vi "S8300E_BARCODE.vi"() -> ()   [LabVIEW 2011]
uses:
  <vilib>/event_ctls.llb/eventvkey.ctl
panel:
  out "軟體版本Software Version":string
  out "begin":u32
  in  "Product SN產品序號":string="192.168.1.3\n192.168.1.1\n192.168.1.1"
  # "輸入條碼上的資訊"
  # "2014-8-21"
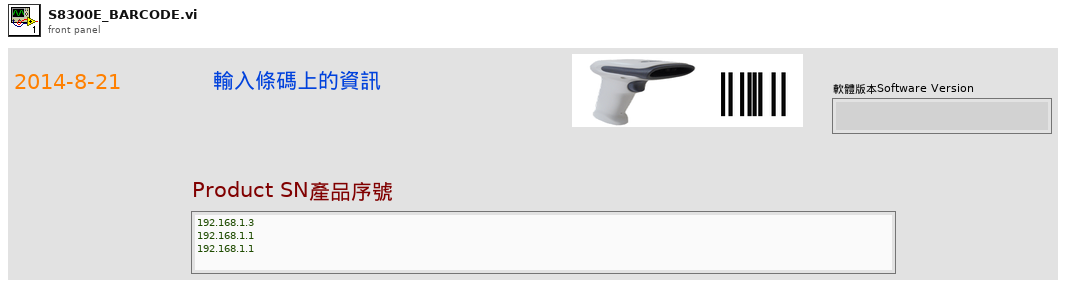
[diagram p1: front panel]
types:
  T1 = typedef "eventvkey.ctl" = enum16{"ASCII", "Enter", "Return", "Shift", "Ctrl", "Alt", "Cmd", "Opt", "Caps", "NumLock", "Clear", "Break", "Up", "Down", "Left", "Right", "Insert", "Delete", "Home", "End", "PageUp", "PageDown", "Escape", "Help", "Pause", "ScrollLock", "F1", "F2", "F3", "F4", "F5", "F6", "F7", "F8", "F9", "F10", "F11", "F12", "F13", "F14", "F15", "F16", "F17", "F18", "F19", "F20", "F21", "F22", "F23", "F24", "Play", "VolumeUp", "VolumeDown", "Mute", "Two Byte Char"}
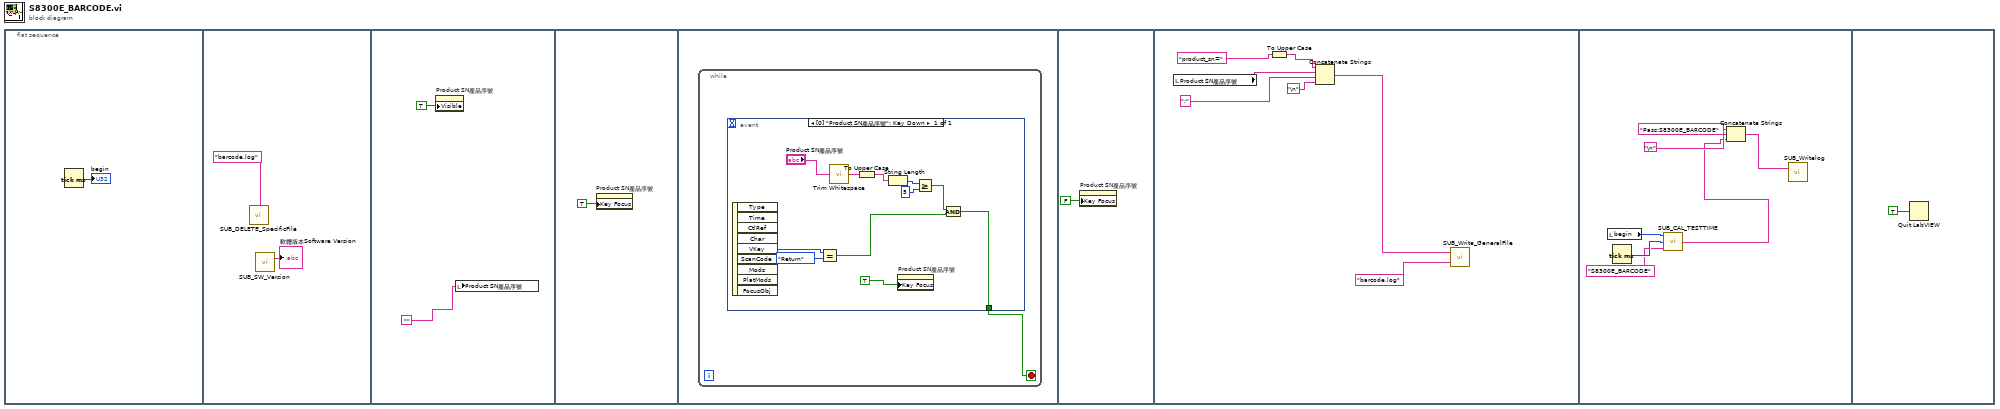
[diagram p0: block diagram]
diagram:
  n1 = flat-sequence {
    frame #0 {
      n2 = Tick Count (ms)() -> (millisecond timer value=→"begin":u32)
    }
    frame #1 {
      n3 = call "SUB_DELETE_SpecificFile.vi"("Filename to be  Deleted"="barcode.log" ("Filename")) -> ()  [unwired: 2 in, 1 out]
      n4 = call "SUB_SW_Version.vi"() -> ("Current Software Version"=→"軟體版本Software Version":string)  [unwired: 3 in]
    }
    frame #2 {
      n5 = property on="Product SN產品序號" class="Str"("Visible"=TRUE) -> ()  [unwired: 2 in, 2 out]
      n6 = local write "Product SN產品序號"("") -> ()
    }
    frame #3 {
      n7 = property on="Product SN產品序號" class="Str"("Key Focus"=TRUE) -> ()  [unwired: 2 in, 2 out]
    }
    frame #4 {
      n8 = while {
        stop <- w7 stop-if-true
        n9 = event shown="[0] \"Product SN產品序號\": Key Down" {
          selector: _ -> [_]
          dyn-events: _ -> [_]
          timeout: _ -> [_]
          tunnel: [w9] -> w7
          event "Product SN產品序號": Key Down {
            n10 = event-data() -> ("VKey"=w12:T1)  [unwired: 1 in, 8 out]
            n11 = Equal?(x=w12, y=eventvkey."Return") -> (x = y?=w10:bool)
            n12 = call <vilib>:"Trim Whitespace.vi"("string"="Product SN產品序號") -> ("trimmed string"=w15:string)  [unwired: 1 in]
            n13 = To Upper Case(1:w15) -> (0:w14:string)
            n14 = String Length(string=w14) -> (length=w18:i32)
            n15 = property on="Product SN產品序號" class="Str"("Key Focus"=TRUE) -> ()  [unwired: 2 in, 2 out]
            n16 = Greater Or Equal?(x=w18, y=5) -> (x >= y?=w16:bool)
            n17 = And(x=w16, y=w10) -> (x .and. y?=w9:bool)
          }
        }
      }
    }
    frame #5 {
      n18 = property on="Product SN產品序號" class="Str"("Key Focus"=FALSE) -> ()  [unwired: 2 in, 2 out]
    }
    frame #6 {
      n19 = local read "Product SN產品序號"() -> (w25:string)
      n20 = To Upper Case(1:"product_sn=" ("string")) -> (0:w21:string)
      n21 = Concatenate Strings(w21, w25, ";", "\n") -> (w20:string)
      n22 = call "SUB_Write_GeneralFile.vi"("Filename"="barcode.log", "Text Input"=w20) -> ()  [unwired: 1 out]
    }
    frame #7 {
      n23 = local read "begin"() -> (w33:u32)
      n24 = Tick Count (ms)() -> (millisecond timer value=w32:u32)
      n25 = call "SUB_CAL_TESTTIME.vi"("Test Item name"="S8300E_BARCODE", "Stop tick time"=w32, "Start tick time"=w33) -> ("Test Time output"=w28:string)  [unwired: 2 in]
      n26 = Concatenate Strings("Pass:S8300E_BARCODE" ("string"), "\n", w28) -> (w27:string)
      n27 = call "SUB_Writelog.vi"("Pass/Fail"=w27) -> ()  [unwired: 2 in]
    }
    frame #8 {
      n28 = Quit LabVIEW(quit? (T)=TRUE) -> ()
    }
  }
